vi "PH_Tektronix_7000.set GUI Refs.vi"(0 "i ref in":refnum<vi>, 2 "Class":string, 3 "GUI Refs":T2, 5 "error in (no error)":errorcluster) -> (14 "i ref out":refnum<vi>, 19 "error out":errorcluster)   [LabVIEW 2014, in "PH_Tektronix_7000.lvlib"]
doc: "This VI is used to set TEKTDS30xx GUI Refs; it shall be used in panels of child classes."
uses:
  PH_Tektronix_7000.lvlib
  PH_Tektronix_7000.GUI Refs.ctl
  PH_Basics/PH_PSDBWriter/PH_PSDBWriter.lvlib
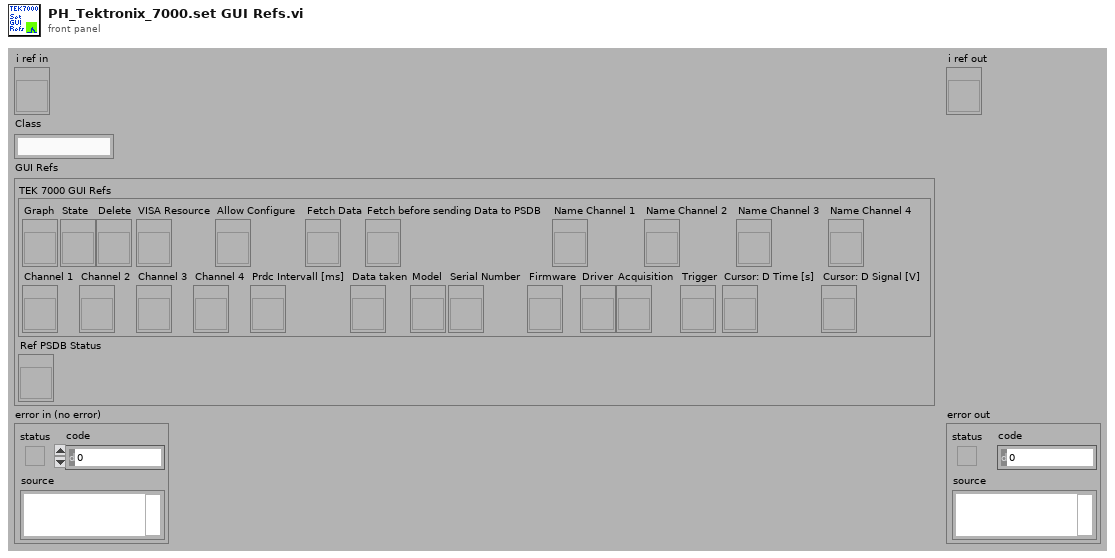
[diagram p1: front panel]
types:
  T1 = typedef "PH_Tektronix_7000.lvlib/PH_Tektronix_7000.GUI Refs.ctl" = cluster{"Graph":refnum<vi>, "State":refnum<vi>, "Delete":refnum<vi>, "VISA Resource":refnum<vi>, "Allow Configure":refnum<vi>, "Fetch Data":refnum<vi>, "Fetch before sending Data to PSDB":refnum<vi>, "Name Channel 1":refnum<vi>, "Name Channel 2":refnum<vi>, "Name Channel 3":refnum<vi>, "Name Channel 4":refnum<vi>, "Prdc Intervall [ms]":refnum<vi>, "Data taken":refnum<vi>, "Model":refnum<vi>, "Serial Number":refnum<vi>, "Firmware":refnum<vi>, "Driver":refnum<vi>, "Acquisition":refnum<vi>, "Trigger":refnum<vi>, "Cursor: D Time [s]":refnum<vi>, "Cursor: D Signal [V]":refnum<vi>, "Channel 1":refnum<vi>, "Channel 2":refnum<vi>, "Channel 3":refnum<vi>, "Channel 4":refnum<vi>}
  T2 = cluster{"TEK 7000 GUI Refs":T1, "Ref PSDB Status":refnum<vi>}
  T3 = typedef "PH_Tektronix_7000.lvlib/PH_Tektronix_7000.i attribute.ctl" = cluster{"VISA Resource Name":refnum<visa-resource-name>, "IDN":cluster{"Instrument Driver":string, "Instrument Firmware":string, "Model":string, "Serial Number":string}, "Selftest":cluster{"Result":i32, "Message":string}, "Trigger Configuration":T4, "Acquisition Configuration":T5, "GUI Refs":T1, "State":T6, "Error Message":string, "Allow Prdc Loop?":bool, "Channel 1":T7, "Channel 2":T7, "Channel 3":T7, "Channel 4":T7, "Data CH 1":waveform(dbl), "Data CH 2":waveform(dbl), "Data CH 3":waveform(dbl), "Data CH 4":waveform(dbl), "Allow config?":bool, "Name Channel 1":string, "Name Channel 2":string, "Name Channel 3":string, "Name Channel 4":string, "Fetch Data before sending to PSDB?":bool, "Constructor passed?":bool, "Data taken at":timestamp, "Plot Colors":u32[], "Default VISA Resource":string}
  T4 = typedef "PH_Tektronix_7000.lvlib/PH_Tektronix_7000.Trigger Config.ctl" = cluster{"Source":u16, "Level [V]":dbl, "Slope":u16, "Coupling":u16, "Trigger Mode":u16}
  T5 = typedef "PH_Tektronix_7000.lvlib/PH_Tektronix_7000.Acquisition Config.ctl" = cluster{"Record Length":u32, "Timebase [s/div]":dbl, "Position [%]":dbl, "Acquisition Type":u16, "Average Waveforms":i32, "Envelope Waveforms":i32, "WfmDB Samples":i32, "Continuous?":bool, "Delay [s]":dbl, "Run?":bool}
  T6 = typedef "PH_StatusHandler.lvlib/PH_StatusHandler.Status.ctl" = i16
  T7 = typedef "PH_Tektronix_7000.lvlib/PH_Tektronix_7000.Channel Config.ctl" = cluster{"Enable Channel":bool, "Bandwidth":u16, "Input Impedance":u16, "Vertical Coupling":u16, "Probe Attenuation":dbl, "Range [V/div]":dbl, "Position [div]":dbl, "Bandwidth raw":string}
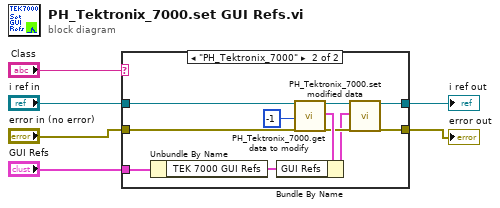
[diagram p0: block diagram]
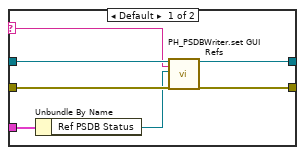
[diagram p2: hidden frame]
diagram:
  n1 = case shown="\"PH_Tektronix_7000\"" "Class" {
    selector: "Class" -> [w9 _]
    tunnel: "error in (no error)" -> [w12 w23]
    tunnel: "i ref in" -> [w13 w22]
    tunnel: [w11 w17] -> w4
    tunnel: [w10 w16] -> w3
    tunnel: "GUI Refs" -> [w8 w15]
    frame Default {
      n2 = Unbundle By Name(w8) -> ("Ref PSDB Status"=w7:refnum<vi>)
      n3 = call "PH_PSDBWriter.set GUI Refs.vi"("i ref in"=w13, "Class"=w9, "Ref PSDB Status"=w7, "error in"=w12) -> ("i ref out"=w11:refnum<vi>, "error out"=w10:errorcluster)  [unwired: 14 in]
    }
    frame "PH_Tektronix_7000" {
      n4 = Unbundle By Name(w15) -> ("TEK 7000 GUI Refs"=w14:T1)
      n5 = call "PH_Tektronix_7000.get data to modify.vi"("i ref in"=w22, "ms timeout (10000)"=-1, "error in (no error)"=w23) -> ("i ref out"=w19:refnum<vi>, "i attribute"=w24:T3, "error out"=w20:errorcluster)  [unwired: 13 in, 1 out]
      n6 = Bundle By Name(cluster=w24, "GUI Refs"=w14) -> (w18:T3)
      n7 = call "PH_Tektronix_7000.set modified data.vi"("i ref in"=w19, "i attribute"=w18, "error in (no error)"=w20) -> ("i ref out"=w17:refnum<vi>, "error out"=w16:errorcluster)  [unwired: 15 in]
    }
  }
  "error out" <- w3
  "i ref out" <- w4
